vi "Write Sub Panel Prod.vi"(8 "error in (no error)":errorcluster, 10 "Sub Panel Prod":refnum<vi>, 11 "Doña Rata Actor in":refnum<class "Doña Rata Actor.lvclass">) -> (0 "error out":errorcluster, 3 "Doña Rata Actor out":refnum<class "Doña Rata Actor.lvclass">)   [LabVIEW 2020, in "Doña Rata Actor.lvlib" / "Doña Rata Actor.lvclass"]
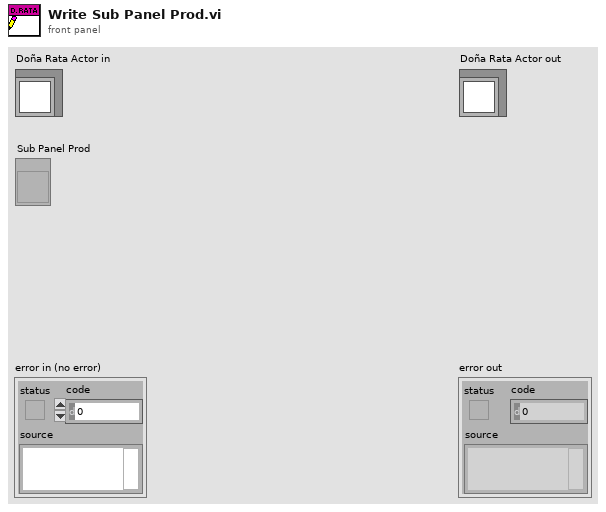
[diagram p1: front panel]
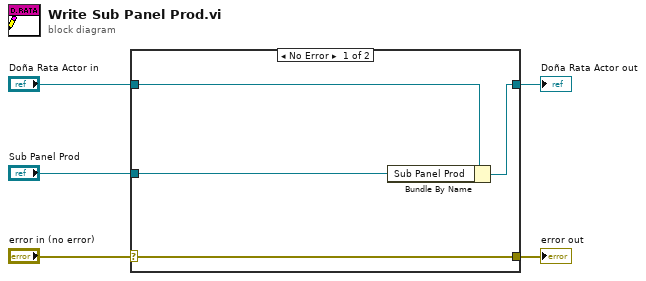
[diagram p0: block diagram]
diagram:
  n1 = case shown="No Error" "error in (no error)" {
    selector: "error in (no error)" -> [w9 w10]
    tunnel: [w9 w10] -> w4
    tunnel: [w7 w11] -> w2
    tunnel: "Doña Rata Actor in" -> [w8 w11]
    tunnel: "Sub Panel Prod" -> [w6 _]
    frame No Error {
      n2 = Bundle By Name(cluster=w8, "Sub Panel Prod"=w6) -> (w7:refnum<class "Doña Rata Actor.lvclass">)
    }
    frame Error {
    }
  }
  "error out" <- w4
  "Doña Rata Actor out" <- w2
